vi "Do Write.vi"(8 "error in (no error)":errorcluster, 9 "Timeout ms":i32, 10 "Data":string, 11 "WebSocket Client in":refnum<class "WebSocket Client.lvclass">) -> (0 "error out":errorcluster, 1 "Remaining  Timeout":i32, 3 "WebSocket Client out":refnum<class "WebSocket Client.lvclass">)   [LabVIEW 2020, in "HTTP Server.lvlib" / "WebSocket Client.lvclass"]
uses:
  WebSocket Client.lvclass
  WebSocket Client.lvclass/WebSocket Client.ctl
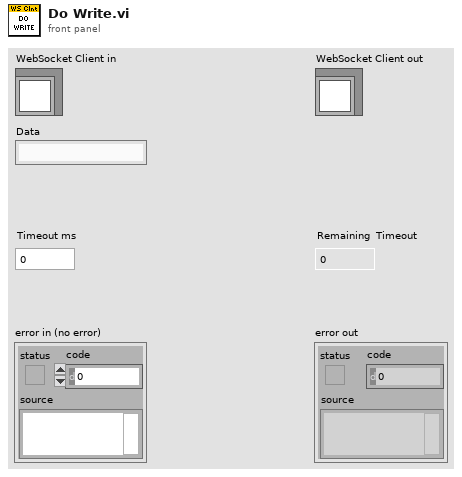
[diagram p1: front panel]
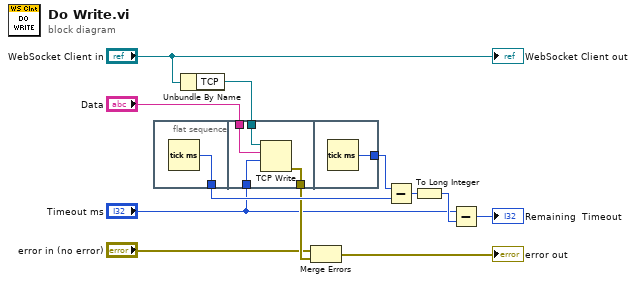
[diagram p0: block diagram]
diagram:
  n1 = flat-sequence {
    tunnel: [w13] -> w10
    tunnel: w12 -> [w17]
    tunnel: "Data" -> [w16]
    tunnel: "Timeout ms" -> [w15]
    tunnel: [w14] -> w7
    tunnel: [w18] -> w11
    frame #0 {
      n2 = Tick Count (ms)() -> (millisecond timer value=w13:u32)
    }
    frame #1 {
      n3 = TCP Write(connection ID=w17, data in=w16, 9:w15) -> (error out=w14:errorcluster)  [unwired: 1 in, 2 out]
    }
    frame #2 {
      n4 = Tick Count (ms)() -> (millisecond timer value=w18:u32)
    }
  }
  n5 = Unbundle By Name("WebSocket Client in") -> ("TCP"=w12:refnum<k5>)
  n6 = Merge Errors("error in (no error)", w7) -> (→"error out":errorcluster)
  n7 = Subtract(x=w11, y=w10) -> (x-y=w9:u32)
  n8 = To Long Integer(number=w9) -> (32bit integer=w8:i32)
  n9 = Subtract(x="Timeout ms", y=w8) -> (x-y=→"Remaining  Timeout":i32)
  "WebSocket Client out" <- "WebSocket Client in"
